vi "T-Vector.vi"() -> (2 "T":u32[](array[numeric]) format="%08x")   [LabVIEW 2013, in "MD5.lvlib" / "MD5.lvclass"]
uses:
  MD5.lvclass
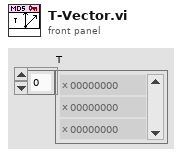
[diagram p1: front panel]
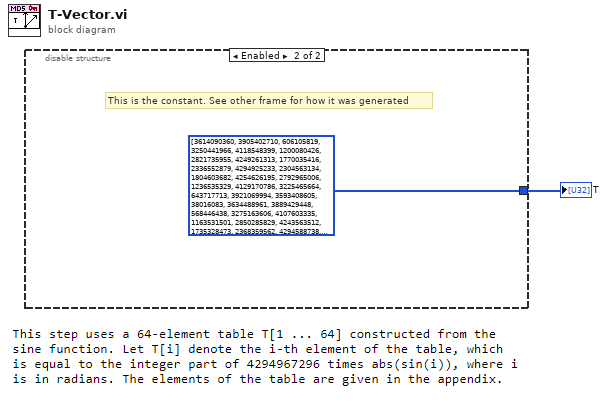
[diagram p0: block diagram]
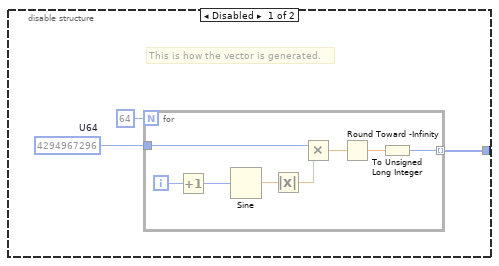
[diagram p2: hidden frame]
diagram:
  n1 = disable-structure shown="Enabled" {
    disable-tunnel: [w2 u32[] [3614090360, 3905402710, 606105819, 3250441966, 4118548399, 1200080426, 2821735955, 4249261313, 1770035416, 2336552879, 4294925233, 2304563134, 1804603682, 4254626195, 2792965006, 1236535329, 4129170786, 3225465664, 643717713, 3921069994, 3593408605, 38016083, 3634488961, 3889429448, 568446438, 3275163606, 4107603335, 1163531501, 2850285829, 4243563512, 1735328473, 2368359562, 4294588738, 2272392833, 1839030562, 4259657740, 2763975236, 1272893353, 4139469664, 3200236656, 681279174, 3936430074, 3572445317, 76029189, 3654602809, 3873151461, 530742520, 3299628645, 4096336452, 1126891415, 2878612391, 4237533241, 1700485571, 2399980690, 4293915773, 2240044497, 1873313359, 4264355552, 2734768916, 1309151649, 4149444226, 3174756917, 718787259, 3951481745] ("T")] -> w1
    frame Disabled {
      w3 = u64 4294967296  # U64
      # "This is how the vector is generated."
      n2 = for {
        N: 64 -> [_]
        tunnel: w3 -> [w10]
        tunnel: [w5] -> w2 mode=indexing
        i -> [w9]
        n3 = Increment(x=w9) -> (x+1=w8:i32)
        n4 = Sine(x=w8) -> (sin(x)=w12:dbl)
        n5 = Absolute Value(x=w12) -> (abs(x)=w11:dbl)
        n6 = Multiply(x=w10, y=w11) -> (x*y=w7:dbl)
        n7 = Round Toward -Infinity(1:w7) -> (0:w6:dbl)
        n8 = To Unsigned Long Integer(number=w6) -> (unsigned 32bit integer=w5:u32)
      }
    }
    frame Enabled {
      # "This is the constant. See other frame for how it was generated"
    }
  }
  "T" <- w1
